vi "PXI Multipliers Notifier.vi"   [LabVIEW 2015]
uses:
  DAQ Engine VIs/PXI Globals.vi
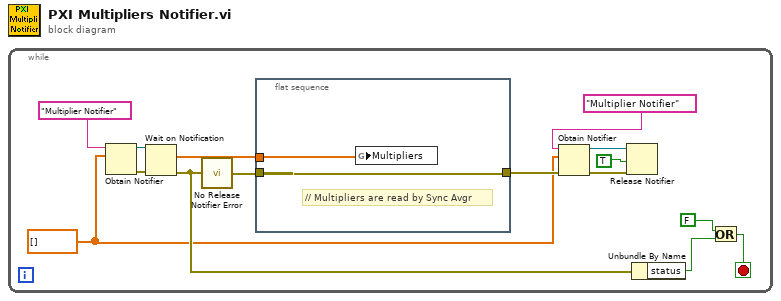
[diagram p0: block diagram]
diagram:
  n1 = while {
    stop <- w2 stop-if-true
    w1 = dbl[] []
    n2 = Obtain Notifier(name (unnamed)="Multiplier Notifier", notification data type=w1) -> (notifier out=w7:refnum<notifier>, error out=w8:errorcluster)  [unwired: 2 in, 1 out]
    n3 = Wait on Notification(notifier=w7, error in (no error)=w8) -> (notification=w9:dbl[], error out=w15:errorcluster)  [unwired: 2 in, 2 out]
    n4 = call "No Release Notifier Error.vi"("error in"=w15) -> ("error out"=w10:errorcluster)  [unwired: 14 in]
    n5 = flat-sequence {
      tunnel: w9 -> [w16]
      tunnel: w10 -> [w17]
      tunnel: [w17] -> w14
      frame #0 {
        # "// Multipliers are read by Sync Avgr"
        n6 = global write "PXI Globals.vi" "Multipliers"(w16) -> ()
      }
    }
    n7 = Obtain Notifier(name (unnamed)="Multiplier Notifier", notification data type=w1, error in (no error)=w14) -> (notifier out=w12:refnum<notifier>, error out=w13:errorcluster)  [unwired: 1 in, 1 out]
    n8 = Release Notifier(notifier=w12, force destroy? (F)=TRUE, error in (no error)=w13) -> ()  [unwired: 3 out]
    n9 = Unbundle By Name(w15) -> ("status"=w3:bool)
    n10 = Or(x=FALSE, y=w3) -> (x .or. y?=w2:bool)
  }
